vi "Pulse Switch Toggle.vi"(0 "Input Switch":bool, 3 "Time/Loop Time":i32) -> (7 "Pulse Switch":bool, 10 "f":i32)   [LabVIEW 2020]
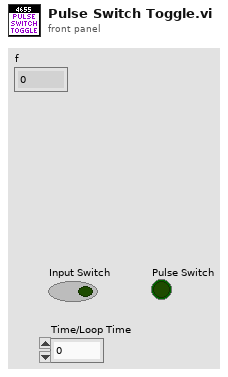
[diagram p1: front panel]
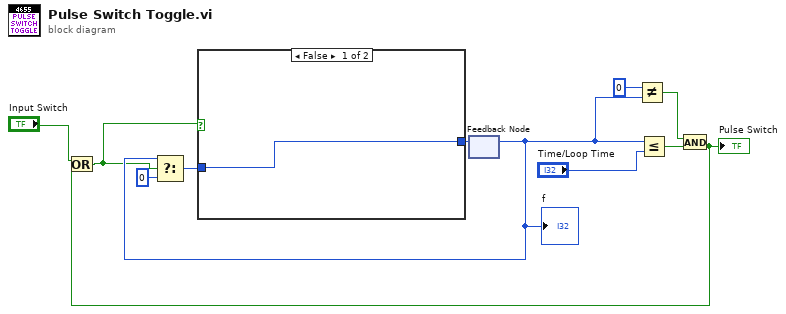
[diagram p0: block diagram]
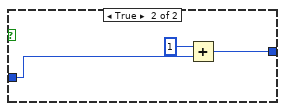
[diagram p2: hidden frame]
diagram:
  n1 = feedback #1() -> (w6:i32)  [unwired: 1 in]
  "f" <- w6
  n2 = Not Equal?(x=0, y=w6) -> (x != y?=w4:bool)
  n3 = Less Or Equal?(x=w6, y="Time/Loop Time") -> (x <= y?=w10:bool)
  n4 = And(x=w4, y=w10) -> (x .and. y?=w2:bool)
  "Pulse Switch" <- w2
  n5 = Or(x="Input Switch", y=w2) -> (x .or. y?=w1:bool)
  n6 = Select(t=w6, s=w1, f=0) -> (s? t:f=w9:i32)
  n7 = case shown="False" w1 {
    tunnel: w9 -> [w12 w15]
    tunnel: [w12 w14] -> w11
    frame False {
    }
    frame True {
      n8 = Add(x=1, y=w15) -> (x+y=w14:i32)
    }
  }
  n9 = feedback-in #1(w11) -> ()
